vi "ShotInterception.vi"(6 "Ally?":bool, 8 "error in (no error)":errorcluster, 9 "Point":dbl[](array[numeric]), 10 "GameRef":refnum<data-value>, 11 "BallInterception in":refnum<class "PassInterception.lvclass">) -> (0 "error out":errorcluster, 2 "Evaluation":dbl, 3 "BallInterception out":refnum<class "PassInterception.lvclass">)   [LabVIEW 2023, in "PassInterception.lvclass"]
uses:
  PassInterception.lvclass
  Game_class/Game.lvclass
  Game_class/Game.lvclass/Game.ctl
  Referee_class/Referee.lvclass/Referee.ctl
  Team_class/Team.lvclass/Team.ctl
  Field_class/Field.lvclass/Field.ctl
  Robot_class/Robot.lvclass/Robot.ctl
  Object_class/Object.lvclass/Object.ctl
  <vilib>/Analysis/coordinate.llb/2D Cartesian Coordinate Shift (Scalar).vi
  <vilib>/Analysis/coordinate.llb/2D Cartesian Coordinate Rotation (Scalar).vi
  Robot_class/Read id.vi
  Object_class/Read position(x,y).vi
  Game_class/Read Referee.vi
  Game_class/Read EnemyRef.vi
  Game_class/Read BallRef.vi
  Game_class/Read Utilities.lvclass.vi
  Game_class/Read FieldRef.vi
  Field_class/Read enemyGoalPosition.vi
  Field_class/Read ourGoalPosition.vi
  Team_class/Read RobotRef.vi
  Referee_class/Read enemy_goalie_id.vi
  Enemy_class/Enemy.lvclass
  C:/Users/ebert/Documents/codes/SSL/repo/SSL_AI/Team_class/Team.lvclass
  Robot_class/Robot.lvclass
  C:/Users/ebert/Documents/codes/SSL/repo/SSL_AI/Object_class/Object.lvclass
  Referee_class/Referee.lvclass
  Ball_class/Ball.lvclass
  Utilities_class/Utilities.lvclass
  Field_class/Field.lvclass
  <vilib>/Analysis/NI_AALPro.lvlib
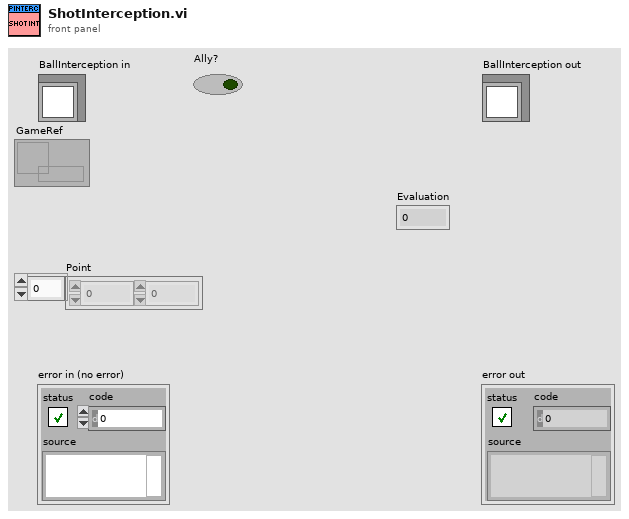
[diagram p1: front panel]
types:
  T1 = typedef "STPParameters.ctl" = cluster{"Skills":T2, "TestSkill":T4, "Events":cluster{"distanceToBallPossession":dbl, "timeForPossessionThreshold":dbl}, "Criteria":cluster{"OpenAngleToGoal":cluster{"minAngle":dbl, "maxAngle":dbl, "minEvaluation":dbl}, "PassDistance":cluster{"maxDistance":dbl, "minDistance":dbl}, "ShotInterception":cluster{"shotSpeed":dbl, "minEnemySpeed":dbl, "minEvaluation":dbl, "maxEnemySpeed":dbl}, "OneTouchShot":cluster{"MaxAngle":dbl, "minEvaluation":dbl}, "PassInterception":cluster{"minEnemySpeed":dbl, "maxEnemySpeed":dbl, "chipPassDistance":dbl, "chipPassEval":dbl, "minEvaluation":dbl}}, "minPassSpeed":dbl, "maxPassSpeed":dbl, "AllyTeamIds":T5[], "ReceiverSpeed":dbl, "minEvaluationToShoot":dbl}
  T2 = typedef "Skills.ctl" = cluster{"CirculateBall":T3, "ProtectBall":cluster{"DistanceFromBall":dbl}}
  T3 = typedef "CIrculateSkillParameters.ctl" = cluster{"rotationAngle":dbl, "velocityFactor":dbl, "OrientationFactor":dbl}
  T4 = typedef "TestSkills.ctl" = enum16{"AlignSkill", "PassSkill", "CirculateBall", "OneTouchShotSkill", "KickToSkill_v2", "ShootSkill", "InterceptBall", "Exit", "GoToSkill_v2"}
  T5 = typedef "AllyTeam.ctl" = enum16{"Keeper", "Defender", "Attacker"}
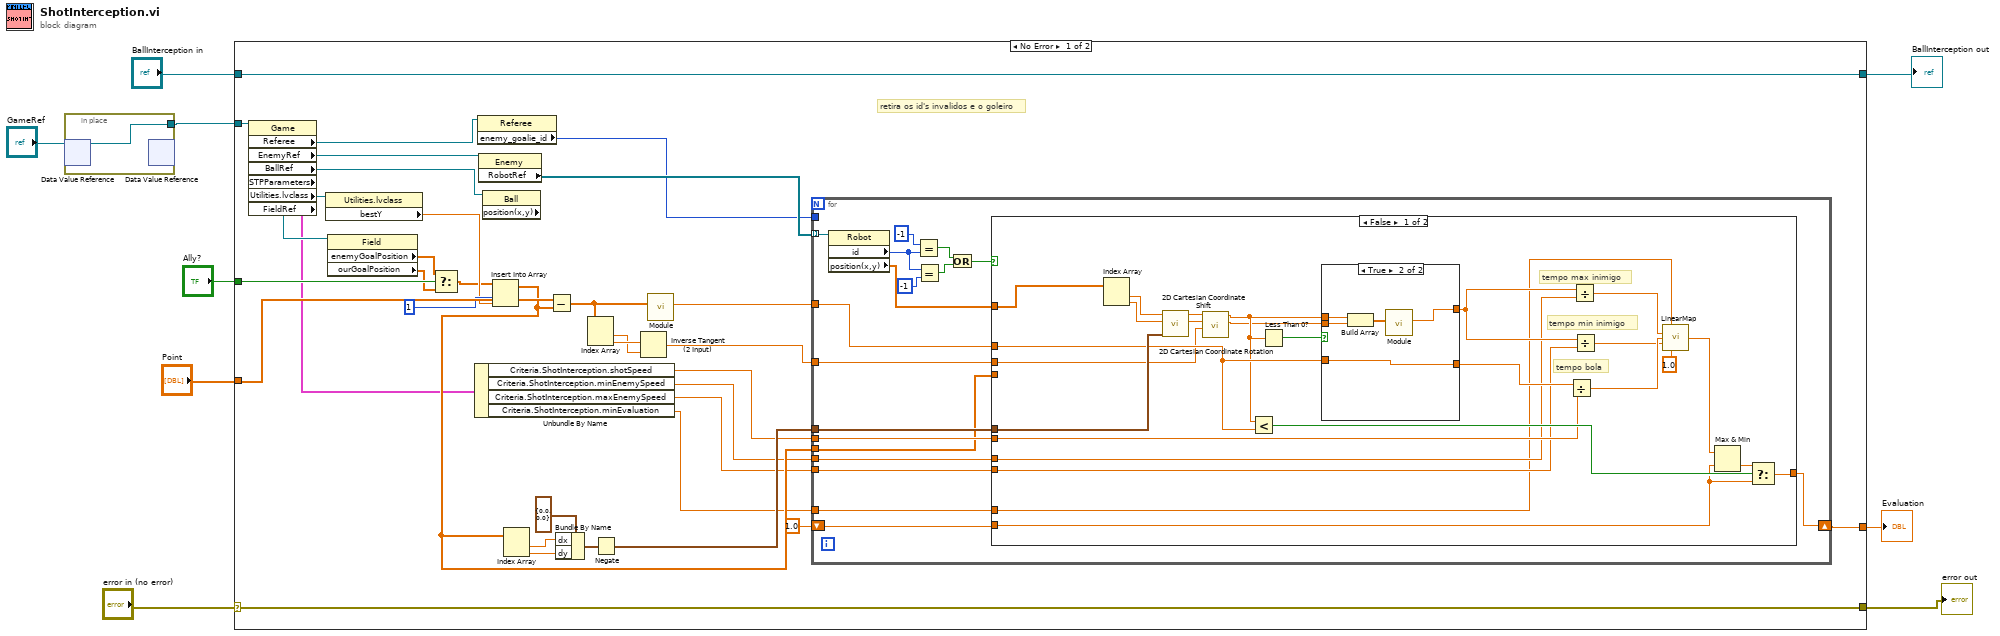
[diagram p0: block diagram]
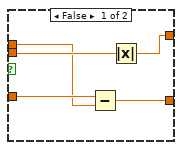
[diagram p2: hidden frame]
diagram:
  n1 = in-place {
    in-place-border: [w10] -> w1
    n2 = in-place-dvr #1("GameRef") -> (w10:refnum<class "Game.lvclass">)  [unwired: 1 out]
    n3 = in-place-dvr #1() -> ()  [unwired: 1 in, 2 out]
  }
  n4 = case shown="No Error" "error in (no error)" {
    selector: "error in (no error)" -> [w45 w102]
    tunnel: [w45 w102] -> w4
    tunnel: "BallInterception in" -> [w44 w101]
    tunnel: [w44 w101] -> w6
    tunnel: w1 -> [w43 _]
    tunnel: "Point" -> [w24 _]
    tunnel: [w28 _] -> w8
    tunnel: "Ally?" -> [w19 _]
    frame No Error {
      # "retira os id's invalidos e o goleiro"
      n5 = property class="Game"(reference=w43) -> ("Referee"=w40:refnum<class "Referee.lvclass">, "EnemyRef"=w42:refnum<class "Enemy.lvclass">, "BallRef"=w38:refnum<class "Ball.lvclass">, "STPParameters"=w15:T1, "Utilities.lvclass"=w25:refnum<class "Utilities.lvclass">, "FieldRef"=w23:refnum<class "Field.lvclass">)  [unwired: 1 in, 2 out]
      n6 = property class="Utilities.lvclass"(reference=w25) -> ("bestY"=w21:dbl)  [unwired: 1 in, 2 out]
      n7 = property class="Field"(reference=w23) -> ("enemyGoalPosition"=w17:dbl[], "ourGoalPosition"=w16:dbl[])  [unwired: 1 in, 2 out]
      n8 = Select(t=w17, s=w19, f=w16) -> (s? t:f=w18:dbl[])
      n9 = Unbundle By Name(w15) -> ("Criteria.ShotInterception.shotSpeed"=w14:dbl, "Criteria.ShotInterception.minEnemySpeed"=w13:dbl, "Criteria.ShotInterception.maxEnemySpeed"=w12:dbl, "Criteria.ShotInterception.minEvaluation"=w11:dbl)
      n10 = property class="Referee"(reference=w40) -> ("enemy_goalie_id"=w39:i32)  [unwired: 1 in, 2 out]
      n11 = property class="Enemy"(reference=w42) -> ("RobotRef"=w41:refnum<class "Robot.lvclass">[])  [unwired: 1 in, 2 out]
      n12 = property class="Ball" props=["position(x,y)"](reference=w38) -> ()  [unwired: 1 in, 3 out]
      n13 = Insert Into Array(array=w18, index=1, new element=w21) -> (w20:dbl[])
      n14 = Index Array(array=w20) -> (element #1=w33:dbl, element #2=w32:dbl)  [unwired: 2 in]
      n15 = Subtract(x=w24, y=w20) -> (x-y=w31:dbl[])
      n16 = Bundle By Name(cluster=cluster{"dx":dbl, "dy":dbl} {"dx"=0.0, "dy"=0.0} ("shift"), "dx"=w33, "dy"=w32) -> (w27:cluster{"dx":dbl, "dy":dbl})
      n17 = Index Array(array=w31) -> (element #1=w36:dbl, element #2=w37:dbl)  [unwired: 2 in]
      n18 = Negate(x=w27) -> (-x=w26:cluster{"dx":dbl, "dy":dbl})
      n19 = Inverse Tangent (2 Input)(1:w36, 2:w37) -> (0:w35:dbl)
      n20 = call "Module.vi"("2D vector"=w31) -> ("Modulo"=w30:dbl)  [unwired: 8 in, 2 out]
      n21 = for {
        tunnel: w41 -> [w62] mode=indexing
        tunnel: w39 -> [_]
        tunnel: w35 -> [w57]
        tunnel: w26 -> [w55]
        tunnel: w30 -> [w54]
        tunnel: w14 -> [w53]
        shift-right: [w51] -> w28
        shift-left: 1.0 ("Numeric") -> [w52]
        tunnel: w20 -> [w50]
        tunnel: w13 -> [w49]
        tunnel: w12 -> [w48]
        tunnel: w11 -> [w47]
        n22 = property class="Robot"(reference=w62) -> ("id"=w61:i32, "position(x,y)"=w56:dbl[])  [unwired: 1 in, 2 out]
        n23 = Equal?(x=-1, y=w61) -> (x = y?=w59:bool)
        n24 = Equal?(x=w61, y=-1) -> (x = y?=w58:bool)
        n25 = Or(x=w59, y=w58) -> (x .or. y?=w63:bool)
        n26 = case shown="False" w63 {
          tunnel: w57 -> [w71 _]
          tunnel: w56 -> [w85 _]
          tunnel: w55 -> [w89 _]
          tunnel: w54 -> [w80 _]
          tunnel: w53 -> [w81 _]
          tunnel: w52 -> [w72 w100]
          tunnel: [w86 w100] -> w51
          tunnel: w50 -> [_ _]
          tunnel: w49 -> [w78 _]
          tunnel: w48 -> [w77 _]
          tunnel: w47 -> [w64 _]
          frame False {
            # "tempo bola"
            # "tempo min inimigo"
            # "tempo max inimigo"
            n27 = Index Array(array=w85) -> (element #1=w70:dbl, element #2=w69:dbl)  [unwired: 2 in]
            n28 = call-poly <vilib>:"2D Cartesian Coordinate Shift.vi"("shift"=w89, "y"=w69, "x"=w70) -> ("y out"=w67:dbl, "x out"=w68:dbl)  [unwired: 6 in, 1 out]
            n29 = call-poly <vilib>:"2D Cartesian Coordinate Rotation.vi"("theta"=w71, "y"=w67, "x"=w68) -> ("y out"=w65:dbl, "x out"=w66:dbl)  [unwired: 6 in, 1 out]
            n30 = Less?(x=w66, y=w80) -> (x < y?=w87:bool)
            n31 = Less Than 0?(x=w66) -> (x < 0?=w88:bool)
            n32 = case shown="True" w88 {
              tunnel: w66 -> [w90 w97]
              tunnel: w65 -> [w93 w95]
              tunnel: [w92 w99] -> w82
              tunnel: w80 -> [w91 w98]
              tunnel: [w94 w98] -> w79
              frame False {
                n33 = Subtract(x=w91, y=w90) -> (x-y=w94:dbl)
                n34 = Absolute Value(x=w93) -> (abs(x)=w92:dbl)
              }
              frame True {
                n35 = Build Array(w97, w95) -> (w96:dbl[])
                n36 = call "Module.vi"("2D vector"=w96) -> ("Modulo"=w99:dbl)  [unwired: 8 in, 2 out]
              }
            }
            n37 = Divide(x=w79, y=w81) -> (x/y=w84:dbl)
            n38 = Divide(x=w82, y=w78) -> (x/y=w76:dbl)
            n39 = Divide(x=w82, y=w77) -> (x/y=w75:dbl)
            n40 = call "LinearMap.vi"("MaxY"=w64, "MaxX"=w76, "X"=w84, "MinX"=w75, "MinY"=1.0) -> ("Y"=w74:dbl)  [unwired: 8 in, 2 out]
            n41 = Max & Min(x=w74, y=w72) -> (min(x,y)=w73:dbl)  [unwired: 1 out]
            n42 = Select(t=w73, s=w87, f=w72) -> (s? t:f=w86:dbl)
          }
          frame True {
          }
        }
      }
    }
    frame Error {
    }
  }
  "error out" <- w4
  "BallInterception out" <- w6
  "Evaluation" <- w8
